vi "Generate Certificate.vi"() -> ()   [LabVIEW 2020, in "Certificate Generation.lvlib"]
doc: "Generates a self-signed CA server certificate and private key file."
uses:
  Certificate Generation.lvlib
  Certificate Info.ctl
  State.ctl
panel:
  in  "Export":bool
  in  "Output Folder":path
  in  "Import":bool
  in  "PFX Password":string
  in  "Generate PFX":bool caption="Generate .pfx certificate (.NET)"
  in  "Generate":bool
  in  "IP Addresses":string[](array[string])
  in  "Add localhost?":bool
  in  "Town":string
  in  "Organisation Name":string
  in  "Country":string(combo)
  in  "Common Name":string
  in  "Validity (days)":i32=3560
  in  "DNS Names":string[](array[string])
  in  "Path to openssl":path=path "C:/Program Files (x86)/National Instruments/Shared/nissl/openssl.exe"
  # "This tool generates a self-signed SSL certificate bundle which can be used for secure TCP (SSL/TLS) connections.\n\nSelf-signed certificates should be used for internal use/testing only. In production environments, a certificate signed by a known certificate authority (CA) should be used to ensure the certifcate can be validated against a trusted source.\n\nIn order for the certificate to be recognised by browsers, it must be manually added to the certificate store as a trusted CA. For information on how to do this see: https://support.globalsign.com/customer/portal/articles/1211541-install-client-digital-certificate---windows-using-chrome"
  # "Adds localhost DNS names and IP addresses to the certificate."
  # "SSL Certificate Generation Utility"
  # "SSL Certificate Generation Utility"
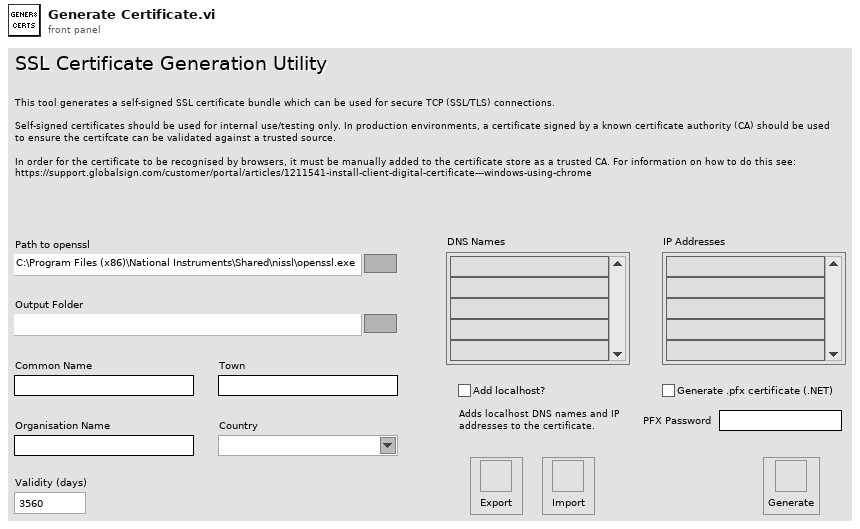
[diagram p1: front panel]
types:
  T1 = typedef "Certificate Generation.lvlib/State.ctl" = enum16{"Initialise", "Handle Events", "Generate Certificate", "Generate PFX", "Exit"}
  T2 = typedef "Certificate Generation.lvlib/Certificate Info.ctl" = cluster{"Common Name":string, "Country":string, "Town":string, "Organisation Name":string, "Alternate DNS Names":string[], "IP Addresses":string[], "Add localhost?":bool, "CA Certificate?":bool}
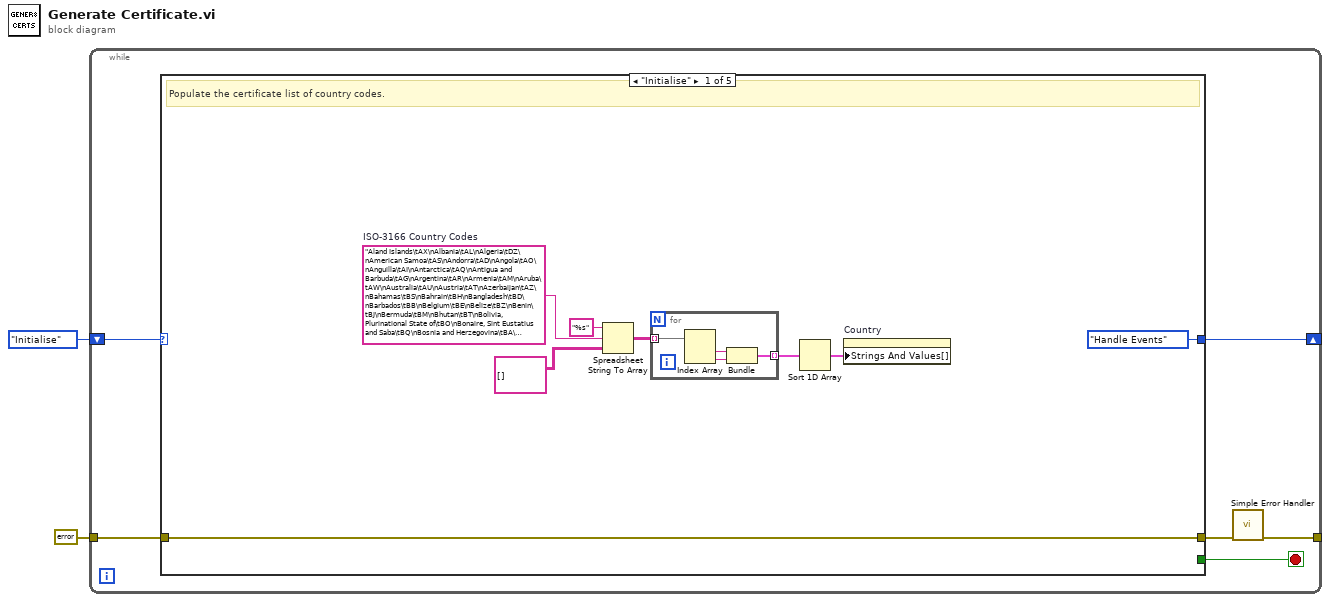
[diagram p0: block diagram]
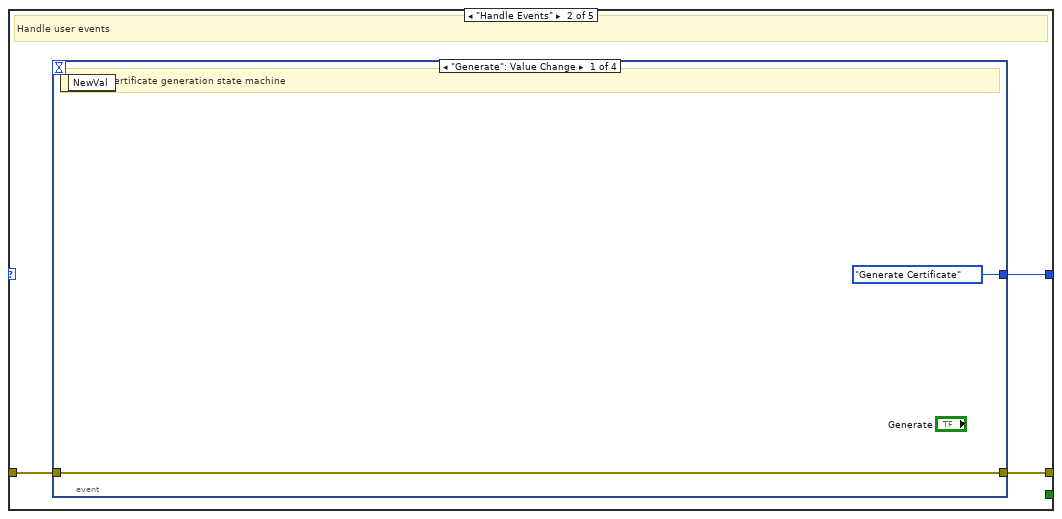
[diagram p2: hidden frame]
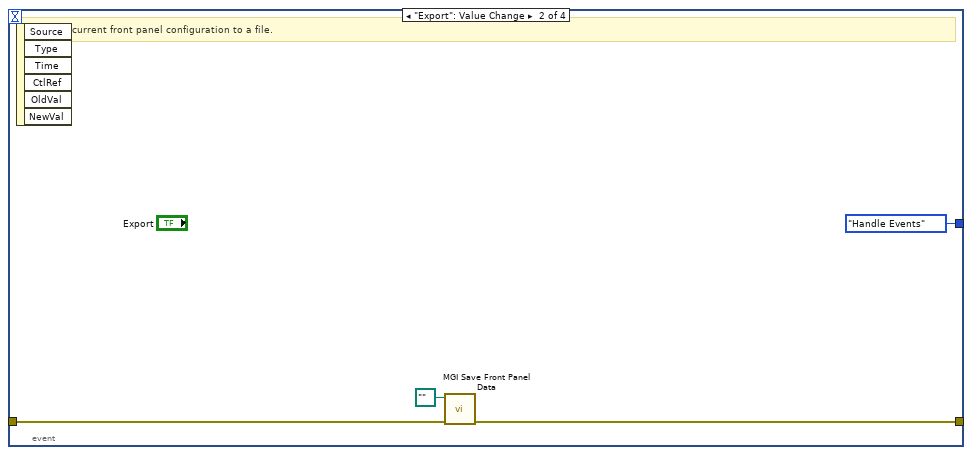
[diagram p3: hidden frame]
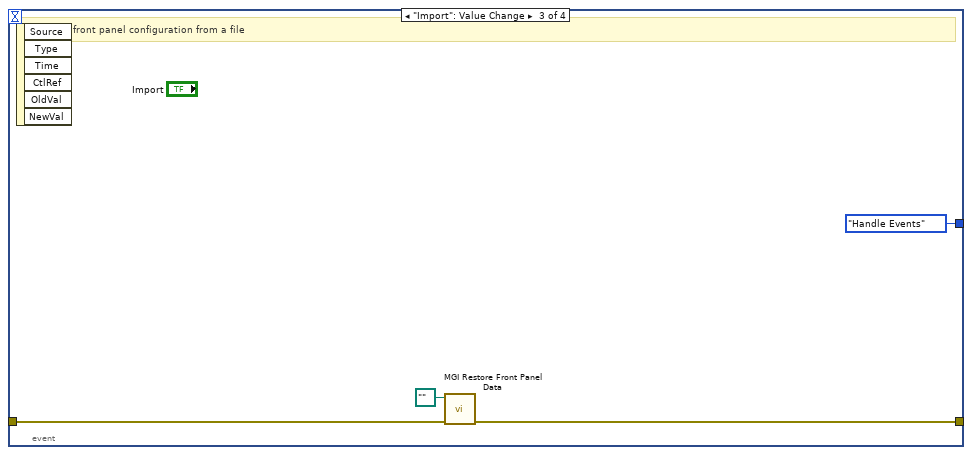
[diagram p4: hidden frame]
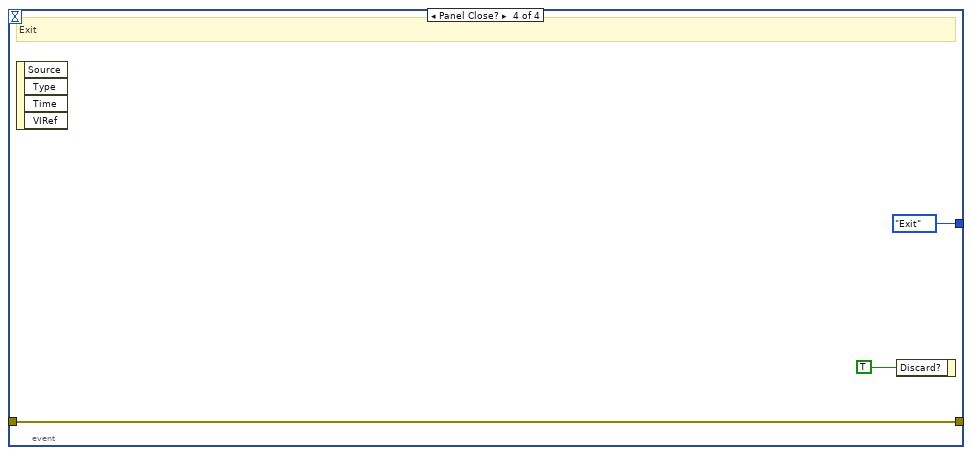
[diagram p5: hidden frame]
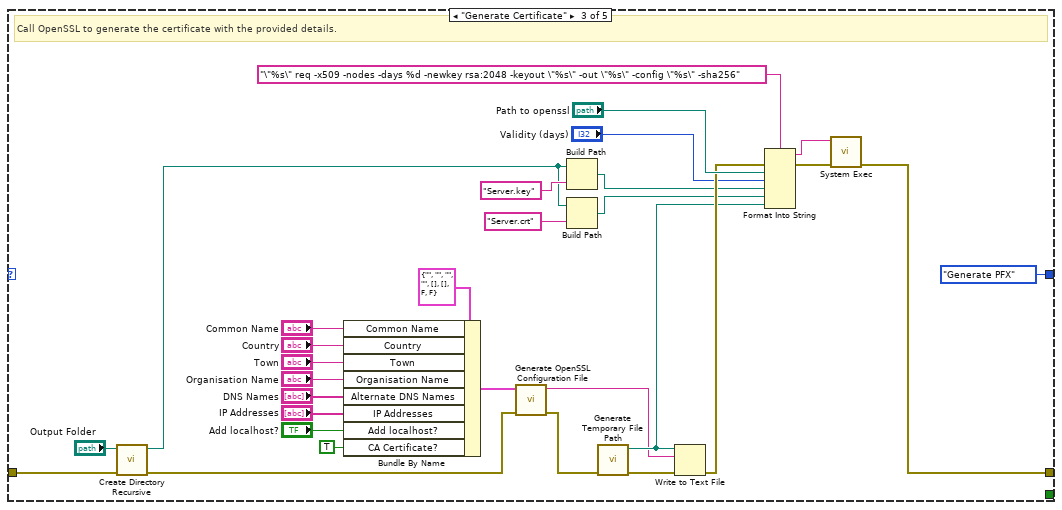
[diagram p6: hidden frame]
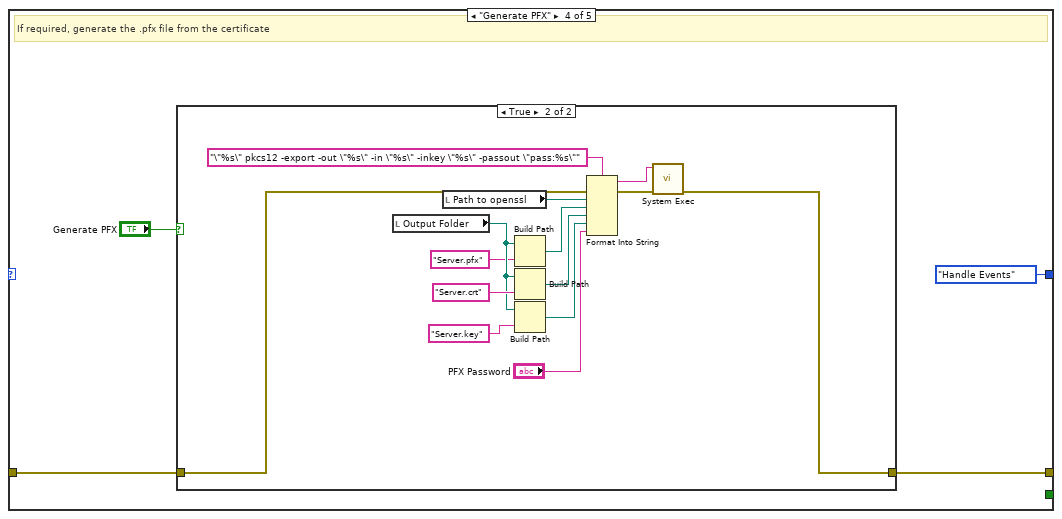
[diagram p7: hidden frame]
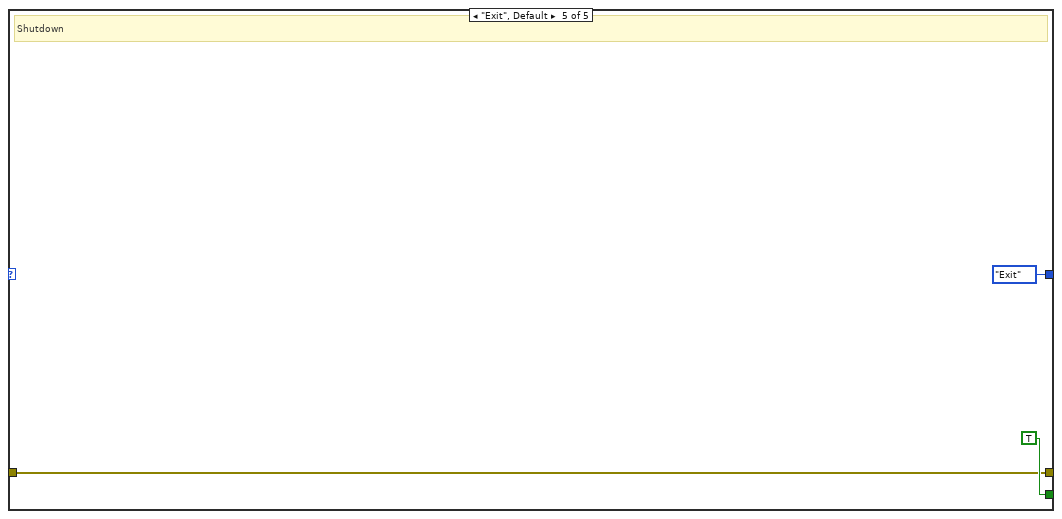
[diagram p9: hidden frame]
diagram:
  n1 = while {
    shift-right: [w6] -> _
    shift-left: State."Initialise" -> [w7]
    tunnel: errorcluster {"status"=FALSE, "code"=0, "source"=""} ("error in (no error)") -> [w4]
    tunnel: [w3] -> _
    stop <- w8 stop-if-true
    n2 = case shown="\"Initialise\"" w7 {
      tunnel: [_ _ _ _ TRUE ("Discard?")] -> w8
      tunnel: [State."Handle Events" w23 State."Generate PFX" State."Handle Events" State."Exit"] -> w6
      tunnel: [w15 w22 w48 w69 w86] -> w5
      tunnel: w4 -> [w15 w21 w38 w68 w86]
      frame "Initialise" {
        w9 = "Aland Islands\tAX\nAlbania\tAL\nAlgeria\tDZ\nAmerican Samoa\tAS\nAndorra\tAD\nAngola\tAO\nAnguilla\tAI\nAntarctica\tAQ\nAntigua and Barbuda\tAG\nArgentina\tAR\nArmenia\tAM\nAruba\tAW\nAustralia\tAU\nAustria\tAT\nAzerbaijan\tAZ\nBahamas\tBS\nBahrain\tBH\nBangladesh\tBD\nBarbados\tBB\nBelgium\tBE\nBelize\tBZ\nBenin\tBJ\nBermuda\tBM\nBhutan\tBT\nBolivia, Plurinational State of\tBO\nBonaire, Sint Eustatius and Saba\tBQ\nBosnia and Herzegovina\tBA\nBotswana\tBW\nBouvet Island\tBV\nBrazil\tBR\nBritish Indian Ocean Territory\tIO\nBrunei Darussalam\tBN\nBulgaria\tBG\nBurkina Faso\tBF\nBurundi\tBI\nCambodia\tKH\nCameroon\tCM\nCanada\tCA\nCape Verde\tCV\nCayman Islands\tKY\nCentral African Republic\tCF\nChad\tTD\nChile\tCL\nChina\tCN\nChristmas Island\tCX\nCocos (Keeling) Islands\tCC\nColombia\tCO\nComoros\tKM\nCongo\tCG\nCongo, Democratic Republic of the\tCD\nCook Islands\tCK\nCosta Rica\tCR\nCroatia\tHR\nCuracao\tCW\nCyprus\tCY\nCzech Republic\tCZ\nDenmark\tDK\nDjibouti\tDJ\nDominica\tDM\nDominican Republic\tDO\nEcuador\tEC\nEgypt\tEG\nEl Salvador\tSV\nEquatorial Guinea\tGQ\nEstonia\tEE\nEthiopia\tET\nFalkland Islands (Malvinas)\tFK\nFaroe Islands\tFO\nFiji\tFJ\nFinland\tFI\nFrance\tFR\nFrench Guiana\tGF\nFrench Polynesia\tPF\nFrench Southern Territories\tTF\nGabon\tGA\nGambia\tGM\nGeorgia\tGE\nGermany\tDE\nGhana\tGH\nGibraltar\tGI\nGreece\tGR\nGreenland\tGL\nGrenada\tGD\nGuadeloupe\tGP\nGuam\tGU\nGuatemala\tGT\nGuernsey\tGG\nGuinea-Bissau\tGW\nGuyana\tGY\nHaiti\tHT\nHeard Island and Mcdonald Islands\tHM\nHoly See (Vatican City State)\tVA\nHonduras\tHN\nHong Kong\tHK\nHungary\tHU\nTokelau\tTK\nTonga\tTO\nTrinidad and Tobago\tTT\nTunisia\tTN\nTurkey\tTR\nTurkmenistan\tTM\nTurks and Caicos Islands\tTC\nTuvalu\tTV\nUganda\tUG\nUkraine\tUA\nUnited Arab Emirates\tAE\nUnited Kingdom\tGB\nUnited States\tUS\nUnited States Minor Outlying Islands\tUM\nUruguay\tUY\nUzbekistan\tUZ\nVanatu\tVU\nVenezuela\tVE\nVietnam\tVN\nVirgin Islands, British\tVG\nVirgin Islands, U.S.\tVI\nWallis and Futuna\tWF\nWestern Sahara\tEH\nYemen\tYE\nZambia\tZM\nAfghanistan\tAF\nBelarus\tBY\nCote D’Ivoire\tCI\nCuba\tCU\nEritrea\tER\nGuinea\tGN\nIran, Islamic Republic of\tIR\nIraq\tIQ\nKorea, Democratic People’s Republic of\tKP\nLebanon\tLB\nLiberia\tLR\nMyanmar\tMM\nPakistan\tPK\nRwanda\tRW\nSierra Leone\tSL\nSouth Sudan\tSS\nSudan\tSD\nSyrian Arab Republic\tSY\nZimbabwe\tZW"  # ISO-3166 Country Codes
        # "Populate the certificate list of country codes."
        n3 = Spreadsheet String To Array(format string="%s", spreadsheet string=w9, array type (2D Dbl)=string[][] []) -> (array=w11:string[][])  [unwired: 1 in]
        n4 = for {
          tunnel: w11 -> [w20] mode=indexing
          tunnel: [w17] -> w12 mode=indexing
          n5 = Index Array(array=w20) -> (element #1=w19:string, element #2=w18:string)  [unwired: 2 in]
          n6 = Bundle(w19, w18) -> (w17:cluster{string, string})  [unwired: 1 in]
        }
        n7 = Sort 1D Array(array=w12) -> (sorted array=w13:cluster{string, string}[])
        n8 = property on="Country" class="CmbBox"("Strings And Values[]"=w13) -> ()  [unwired: 2 in, 2 out]
      }
      frame "Handle Events" {
        # "Handle user events"
        n9 = event shown="[0] \"Generate\": Value Change" {
          selector: _ -> [_ _ _ _]
          dyn-events: _ -> [_ _ _ _]
          timeout: _ -> [_ _ _ _]
          tunnel: [State."Generate Certificate" State."Handle Events" State."Handle Events" State."Exit"] -> w23
          tunnel: [w24 w28 w32 w34] -> w22
          tunnel: w21 -> [w24 w29 w33 w34]
          event "Generate": Value Change {
            # "Start the certificate generation state machine"
            n10 = event-data() -> ()  [unwired: 1 in, 1 out]
          }
          event "Export": Value Change {
            # "Export the current front panel configuration to a file."
            n11 = event-data() -> ()  [unwired: 1 in, 6 out]
            n12 = call <userlib>:"MGI Save Front Panel Data.vi"("error in (no error)"=w29, "Path"=path "") -> ("Error Out"=w28:errorcluster)  [unwired: 9 in]
          }
          event "Import": Value Change {
            # "Import the front panel configuration from a file"
            n13 = event-data() -> ()  [unwired: 1 in, 6 out]
            n14 = call <userlib>:"MGI Restore Front Panel Data.vi"("error in (no error)"=w33, "Path"=path "") -> ("Error Out"=w32:errorcluster)  [unwired: 9 in]
          }
          event Panel Close? {
            # "Exit"
            n15 = event-data() -> ()  [unwired: 1 in, 4 out]
            n16 = event-data("Discard?"=TRUE) -> ()  [unwired: 1 in, 1 out]
          }
        }
      }
      frame "Generate Certificate" {
        # "Call OpenSSL to generate the certificate with the provided details."
        n17 = call <vilib>:"Create Directory Recursive.vi"("error in (no error)"=w38, "directory"="Output Folder") -> ("error out"=w37:errorcluster, "directory copy"=w39:path)  [unwired: 3 in, 1 out]
        n18 = Bundle By Name(cluster=T2 {"Common Name"="", "Country"="", "Town"="", "Organisation Name"="", "Alternate DNS Names"=[], "IP Addresses"=[], "Add localhost?"=FALSE, "CA Certificate?"=FALSE}, "Common Name"="Common Name", "Country"="Country", "Town"="Town", "Organisation Name"="Organisation Name", "Alternate DNS Names"="DNS Names", "IP Addresses"="IP Addresses", "Add localhost?"="Add localhost?", "CA Certificate?"=TRUE) -> (w58:T2)
        n19 = call "Generate OpenSSL Configuration File.vi"("error in (no error)"=w37, "Cert Info"=w58) -> ("error out"=w45:errorcluster, "OpenSSL Cert Config File"=w57:string)  [unwired: 8 in]
        n20 = Build Path(base path=w39, name or relative path="Server.key") -> (appended path=w42:path)
        n21 = Build Path(base path=w39, name or relative path="Server.crt") -> (appended path=w41:path)
        n22 = call <vilib>:"Generate Temporary File Path.vi"("error in (no error)"=w45) -> ("error out"=w64:errorcluster, "Unique Temporary File Path"=w61:path)  [unwired: 9 in]
        n23 = Write to Text File(file (use dialog)=w61, text=w57, error in=w64) -> (error out=w63:errorcluster)  [unwired: 1 in, 2 out]
        n24 = Format Into String(format string="\"%s\" req -x509 -nodes -days %d -newkey rsa:2048 -keyout \"%s\" -out \"%s\" -config \"%s\" -sha256", error in=w63, "Path to openssl", "Validity (days)", w42, w41, w61) -> (resulting string=w62:string, error out=w47:errorcluster)  [unwired: 1 in]
        n25 = call <vilib>:"System Exec.vi"("error in (no error)"=w47, "command line"=w62) -> ("error out"=w48:errorcluster)  [unwired: 6 in, 3 out]
      }
      frame "Generate PFX" {
        # "If required, generate the .pfx file from the certificate"
        n26 = case shown="True" "Generate PFX" {
          tunnel: [w71 w75] -> w69
          tunnel: w68 -> [w71 w74]
          frame False {
          }
          frame True {
            n27 = local read "Output Folder"() -> (w80:path)
            n28 = local read "Path to openssl"() -> (w81:path)
            n29 = Build Path(base path=w80, name or relative path="Server.pfx") -> (appended path=w78:path)
            n30 = Build Path(base path=w80, name or relative path="Server.crt") -> (appended path=w73:path)
            n31 = Build Path(base path=w80, name or relative path="Server.key") -> (appended path=w72:path)
            n32 = Format Into String(format string="\"%s\" pkcs12 -export -out \"%s\" -in \"%s\" -inkey \"%s\" -passout \"pass:%s\"", error in=w74, w81, w78, w73, w72, "PFX Password") -> (resulting string=w76:string, error out=w84:errorcluster)  [unwired: 1 in]
            n33 = call <vilib>:"System Exec.vi"("error in (no error)"=w84, "command line"=w76) -> ("error out"=w75:errorcluster)  [unwired: 6 in, 3 out]
          }
        }
      }
      frame "Exit", Default {
        # "Shutdown"
      }
    }
    n34 = call <vilib>:"Simple Error Handler.vi"("error in (no error)"=w5) -> ("error out"=w3:errorcluster)  [unwired: 4 in, 4 out]
  }
